vi "Write Hardware Handles.vi"(8 "error in":errorcluster, 10 "hardware handles":T1, 11 "Ballard ARINC-429 shared resources in":refnum<class "Ballard ARINC-429 Shared Resources.lvclass">) -> (0 "error out":errorcluster, 3 "Ballard ARINC-429 shared resources out":refnum<class "Ballard ARINC-429 Shared Resources.lvclass">)   [LabVIEW 2020, in "Ballard ARINC 429 Engine.lvlib" / "Implementation.lvlib" / "Ballard ARINC-429 Shared Resources.lvclass"]
uses:
  Ballard ARINC-429 Shared Resources.lvclass
  Custom Device/Hardware Handles.ctl
  Ballard ARINC-429 Shared Resources.lvclass/Ballard ARINC-429 Shared Resources.ctl
  Custom Device/Custom Device.lvlib
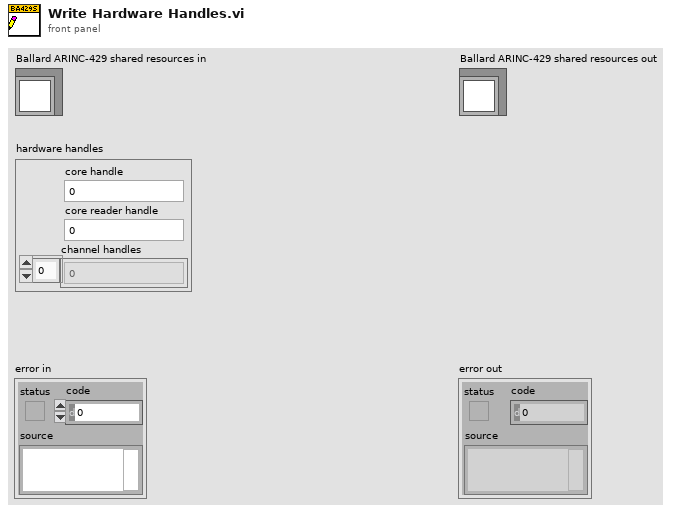
[diagram p1: front panel]
types:
  T1 = typedef "Ballard ARINC 429 Engine.lvlib/Custom Device.lvlib/Hardware Handles.ctl" = cluster{"core handle":u64, "core reader handle":u64, "channel handles":u64[]}
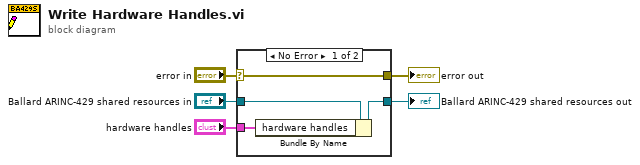
[diagram p0: block diagram]
diagram:
  n1 = case shown="No Error" "error in" {
    selector: "error in" -> [w9 w10]
    tunnel: [w9 w10] -> w4
    tunnel: [w6 w11] -> w2
    tunnel: "Ballard ARINC-429 shared resources in" -> [w8 w11]
    tunnel: "hardware handles" -> [w7 _]
    frame No Error {
      n2 = Bundle By Name(cluster=w8, "hardware handles"=w7) -> (w6:refnum<class "Ballard ARINC-429 Shared Resources.lvclass">)
    }
    frame Error {
    }
  }
  "error out" <- w4
  "Ballard ARINC-429 shared resources out" <- w2
